vi "LabVIEWToPythonImage.vi"(8 "error in (no error)":errorcluster, 10 "image":picture) -> (0 "error out":errorcluster, 2 "Python Image Data":u8[][][](array[numeric]))   [LabVIEW 2017, in "ImageFacialDetection.lvclass"]
doc: "Converts a LabVIEW 2D picture to a Python image - a 3D array with\ndimensions (height, width, color)."
uses:
  ImageFacialDetection.lvclass
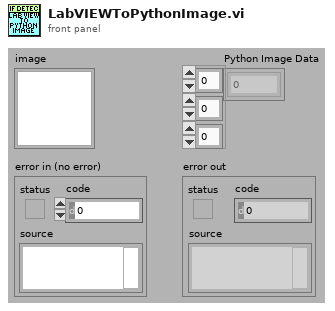
[diagram p1: front panel]
types:
  T1 = typedef "imagedata.ctl" = cluster{"image type":i32, "image depth":i32, "image":u8[], "mask":u8[], "colors":u32[], "Rectangle":cluster{"left":i16, "top":i16, "right":i16, "bottom":i16}}
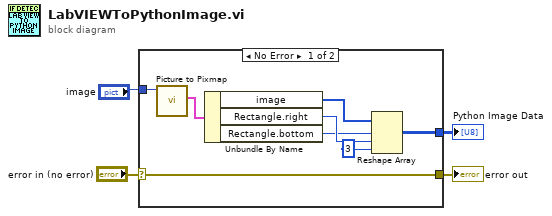
[diagram p0: block diagram]
diagram:
  n1 = case shown="No Error" "error in (no error)" {
    selector: "error in (no error)" -> [w12 w13]
    tunnel: [w12 w13] -> w3
    tunnel: "image" -> [w7 _]
    tunnel: [w5 _] -> w1
    frame No Error {
      n2 = call <vilib>:"Picture to Pixmap.vi"("picture"=w7) -> ("image data"=w6:T1)  [unwired: 9 in, 1 out]
      n3 = Unbundle By Name(w6) -> ("image"=w11:u8[], "Rectangle.right"=w9:i16, "Rectangle.bottom"=w8:i16)
      n4 = Reshape Array(w11, w8, w9, 3 ("dimension size")) -> (w5:u8[][][])
    }
    frame Error {
    }
  }
  "error out" <- w3
  "Python Image Data" <- w1
